vi "Read_from_OPC.vi"() -> ()   [LabVIEW 2021]
panel:
  in  "Toggle logging":bool=TRUE
  out "Temperature":dbl
  in  "stop":bool
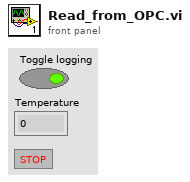
[diagram p1: front panel]
types:
  T1 = enum16{"Read", "Write", "ReadWrite", "BufferedRead", "BufferedReadWrite"}
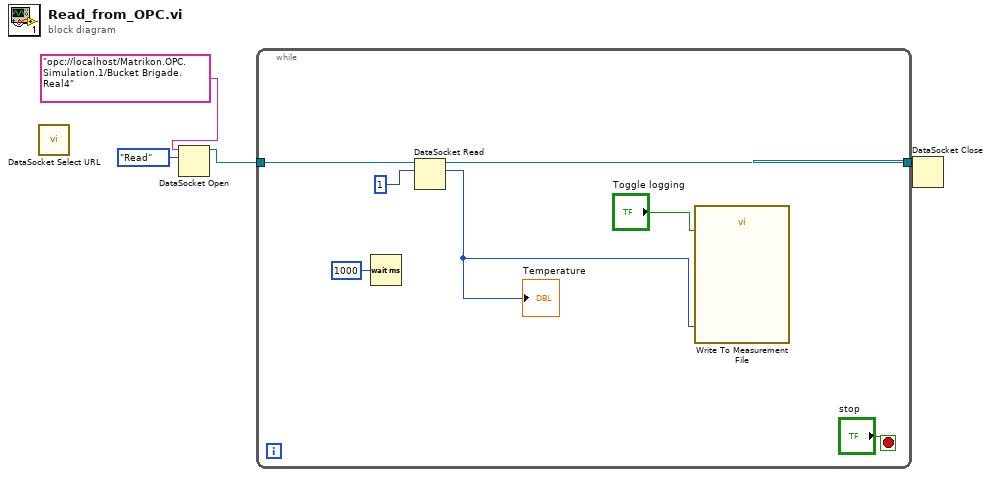
[diagram p0: block diagram]
diagram:
  n1 = call <vilib>:"DataSocket Select URL.vi"() -> ()  [unwired: 9 in, 3 out]
  n2 = DataSocket Open(10:T1."Read" ("mode"), 11:"opc://localhost/Matrikon.OPC.Simulation.1/Bucket Brigade.Real4") -> (3:w3:refnum<k13>)  [unwired: 2 in, 1 out]
  n3 = while {
    tunnel: w3 -> [w9]
    tunnel: [w8] -> w2
    stop <- "stop" stop-if-true
    n4 = Wait (ms)(milliseconds to wait=u32 1000) -> ()  [unwired: 1 out]
    n5 = DataSocket Read(10:u32 1 ("milliseconds to wait"), 11:w9) -> (2:w5:u32, 3:w8:refnum<k13>)  [unwired: 3 in, 5 out]
    "Temperature" <- w5
    n6 = call "Write To Measurement File"("Signals"=w5, "Enable"="Toggle logging") -> ()  [unwired: 15 in, 3 out]
  }
  n7 = DataSocket Close(11:w2) -> ()  [unwired: 2 in, 2 out]
